vi "Labspec GetValue.vi"(6 "Control Refnum":refnum<vi>, 8 "error in":errorcluster, 9 "GetValue Mode":T1, 10 "DataID":i32, 11 "Automation Refnum In":refnum<k7>) -> (0 "error out":errorcluster, 1 "pValue":variant, 3 "Automation Refnum Out":refnum<k7>)   [LabVIEW 2014]
uses:
  GetValue Mode.ctl
panel:
  # "LICENSED MATERIALS – PROPERTY OF IBM\nCopyright IBM Corp. 2016,\nALL RIGHTS RESERVED"
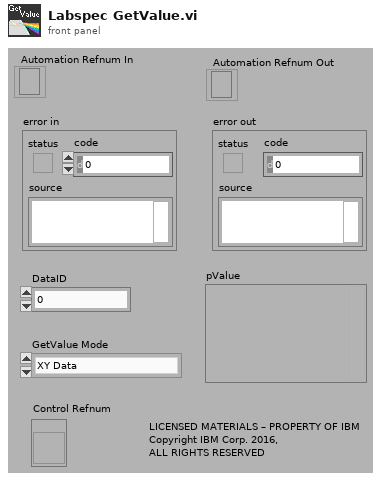
[diagram p1: front panel]
types:
  T1 = typedef "GetValue Mode.ctl" = enum16{"XY Data", "Data", "MapPoint: Spectrum Index", "Axis Labels", "Axis Units", "Axis", "Axis Index", "Axis Size", "Axis Type", "Intensity", "Frequency", "X", "Y", "Z", "Time", "Double Cursor", "Pointer Limits", "Active Cursors", "Nearest Axis Index", "Acquisition Information", "Custom Information", "History Information", "Data Name", "Dispersion", "Dispersion Parameters", "Labspec Path", "User Level", "System Name", "Autofocus Diode", "Exposure Time", "Live Time", "Labspec Accumulation", "Alignment Diode"}
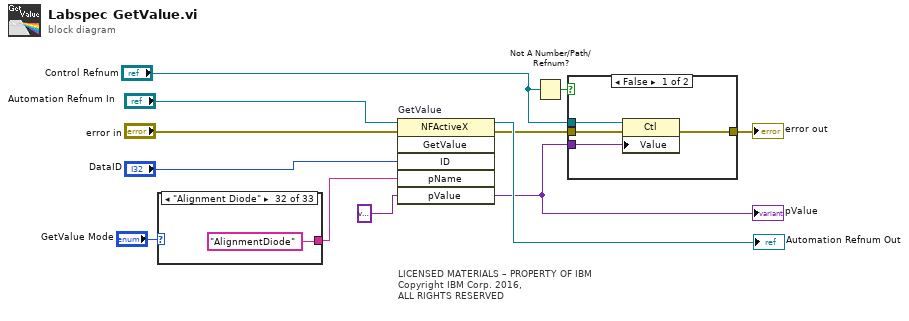
[diagram p0: block diagram]
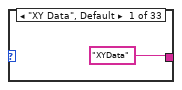
[diagram p3: hidden frame]
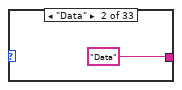
[diagram p4: hidden frame]
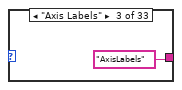
[diagram p5: hidden frame]
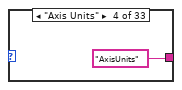
[diagram p6: hidden frame]
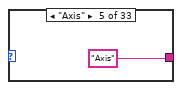
[diagram p7: hidden frame]
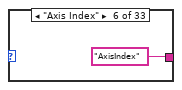
[diagram p8: hidden frame]
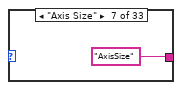
[diagram p9: hidden frame]
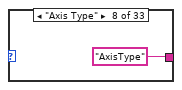
[diagram p10: hidden frame]
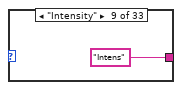
[diagram p11: hidden frame]
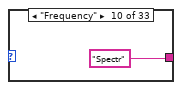
[diagram p12: hidden frame]
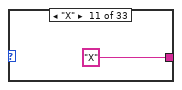
[diagram p13: hidden frame]
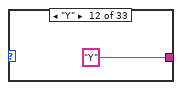
[diagram p14: hidden frame]
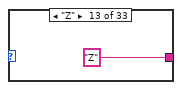
[diagram p15: hidden frame]
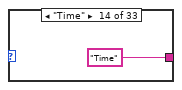
[diagram p16: hidden frame]
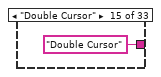
[diagram p17: hidden frame]
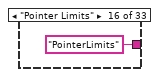
[diagram p18: hidden frame]
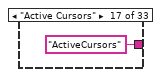
[diagram p19: hidden frame]
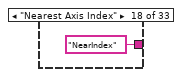
[diagram p20: hidden frame]
diagram:
  # "LICENSED MATERIALS – PROPERTY OF IBM\nCopyright IBM Corp. 2016,\nALL RIGHTS RESERVED"
  n1 = case shown="\"Alignment Diode\"" "GetValue Mode" {
    tunnel: ["XYData" "Data" "AxisLabels" "AxisUnits" "Axis" "AxisIndex" "AxisSize" "AxisType" "Intens" "Spectr" "X" "Y" "Z" "Time" "Double Cursor" "PointerLimits" "ActiveCursors" "NearIndex" "AcqInfo" "CustomInfo" "HistoryInfo" "DataName" "Dispersion" "DispersionParams" "LabSpecPath" "UserLevel" "SystemName" "AutofocusDiode" "LabSpecExposureTime" "LabSpecLiveTime" "LabSpecAccumulation" "AlignmentDiode" "MapPoint:SpectrumIndex"] -> w7
    frame "XY Data", Default {
    }
    frame "Data" {
    }
    frame "Axis Labels" {
    }
    frame "Axis Units" {
    }
    frame "Axis" {
    }
    frame "Axis Index" {
    }
    frame "Axis Size" {
    }
    frame "Axis Type" {
    }
    frame "Intensity" {
    }
    frame "Frequency" {
    }
    frame "X" {
    }
    frame "Y" {
    }
    frame "Z" {
    }
    frame "Time" {
    }
    frame "Double Cursor" {
    }
    frame "Pointer Limits" {
    }
    frame "Active Cursors" {
    }
    frame "Nearest Axis Index" {
    }
    frame "Acquisition Information" {
    }
    frame "Custom Information" {
    }
    frame "History Information" {
    }
    frame "Data Name" {
    }
    frame "Dispersion" {
    }
    frame "Dispersion Parameters" {
    }
    frame "Labspec Path" {
    }
    frame "User Level" {
    }
    frame "System Name" {
    }
    frame "Autofocus Diode" {
    }
    frame "Exposure Time" {
    }
    frame "Live Time" {
    }
    frame "Labspec Accumulation" {
    }
    frame "Alignment Diode" {
    }
    frame "MapPoint: Spectrum Index" {
    }
  }
  n2 = invoke on="GetValue" class="NFActiveX" method="GetValue"(reference="Automation Refnum In", error in="error in", "ID"="DataID", "pName"=w7, "pValue"=variant ("pValue 2")) -> (reference out=→"Automation Refnum Out":refnum<k7>, error out=w2:errorcluster, "pValue"=w3:variant)  [unwired: 1 in, 3 out]
  "pValue" <- w3
  n3 = Not A Number/Path/Refnum?(number/path/refnum="Control Refnum") -> (NaN/Path/Refnum?=w5:bool)
  n4 = case shown="False" w5 {
    tunnel: "Control Refnum" -> [w49 _]
    tunnel: w2 -> [w48 w50]
    tunnel: [w47 w50] -> w1
    tunnel: w3 -> [w46 _]
    frame False {
      n5 = property class="Ctl"(reference=w49, error in=w48, "Value"=w46) -> (error out=w47:errorcluster)  [unwired: 1 out]
    }
    frame True {
    }
  }
  "error out" <- w1
